vi "arms in.vi"(6 "Synchronication":enum16{"Start", "Wait"}(ring), 7 "Description":string, 8 "Command Info In":T1) -> (0 "Command Info Out":T1)   [LabVIEW 2016]
uses:
  <vilib>/Rock Robotics/WPI/Framework/Command Status Info.ctl
  <vilib>/Rock Robotics/WPI/Framework/Completion Status.ctl
  <vilib>/Rock Robotics/WPI/Framework/Completion Notifier.ctl
  Implementation/Gear Setpoints.ctl
  Implementation/Gear Operations.ctl
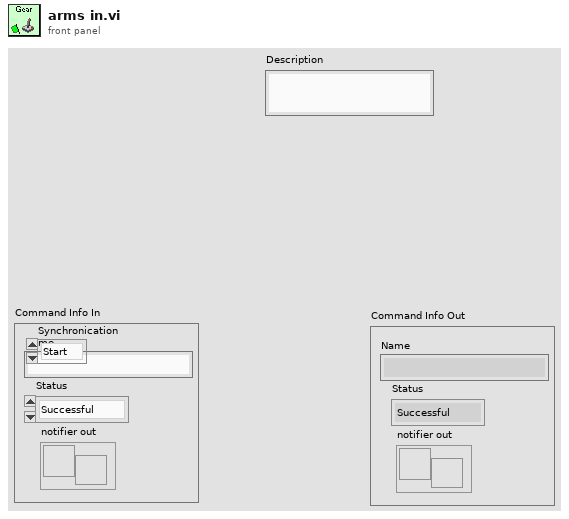
[diagram p1: front panel]
types:
  T1 = typedef "Command Status Info.ctl" = cluster{"Name":string, "Status":T2, "notifier out":T3}
  T2 = typedef "Completion Status.ctl" = enum16{"Successful", "Aborted", "Incomplete"}
  T3 = typedef "Completion Notifier.ctl" = refnum<notifier>
  T4 = typedef "Gear Setpoints.ctl" = cluster{"Operation":T5, "Setpoint":dbl, "Duration":dbl}
  T5 = typedef "Gear Operations.ctl" = enum16{"Reserve", "Read Current", "Immediate", "Go to Scoring", "Go to Intake", "Arms out", "Spin rollers", "Arms in"}
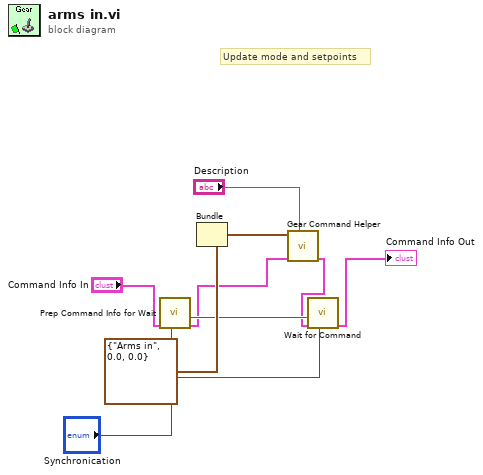
[diagram p0: block diagram]
diagram:
  # "Update mode and setpoints"
  n1 = call <vilib>:"Prep Command Info for Wait.vi"("Synchronication"="Synchronication", "Command Info"="Command Info In") -> ("Command Info"=w3:T1, "Allocated"=w6:bool)  [unwired: 8 in]
  n2 = Bundle(cluster=T4 {"Operation"=enum."Arms in", "Setpoint"=0.0, "Duration"=0.0} ("SubSystem Data")) -> (w7:T4)  [unwired: 3 in]
  n3 = call "Gear Command Helper.vi"("Description"="Description", "Command Info In"=w3, "SubSystem Data"=w7) -> ("Command Info Out"=w2:T1)  [unwired: 7 in, 1 out]
  n4 = call <vilib>:"Wait for Command.vi"("Synchronication"="Synchronication", "Command Info in"=w2, "Allocated"=w6) -> ("Command Info out"=→"Command Info Out":T1)  [unwired: 8 in]
